vi "odometry_msg.vi"(11 "odometry_msg in":string) -> (2 "Current_Pose":T1, 3 "robot_position_cluster":T2)   [LabVIEW 2014]
uses:
  Robot_Position.ctl
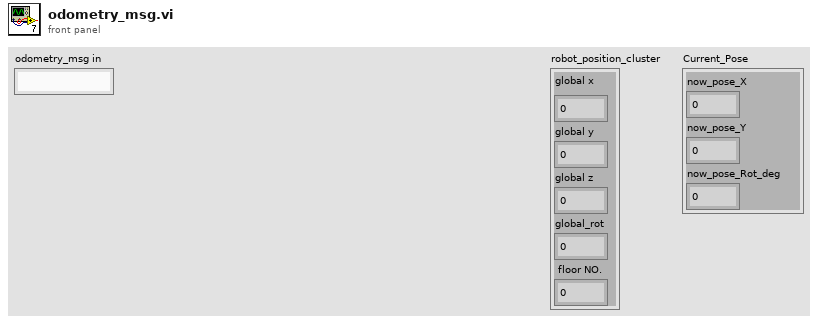
[diagram p1: front panel]
types:
  T1 = cluster{"now_pose_X":dbl, "now_pose_Y":dbl, "now_pose_Rot_deg":dbl}
  T2 = typedef "Robot_Position.ctl" = cluster{"global x":dbl, "global y":dbl, "global z":dbl, "global_rot":dbl, " floor NO.":dbl}
  T3 = cluster{"PoseCovariance":cluster{"Pose":cluster{"Point":cluster{"x":dbl, "y":dbl, "z":dbl}, "Quaternion":cluster{"x":dbl, "y":dbl, "z":dbl, "w":dbl}}, "Covariance":dbl}, "TwistCovariance":cluster{"Twist":cluster{"Linear":cluster{"x":dbl, "y":dbl, "z":dbl}, "Angular":cluster{"x":dbl, "y":dbl, "z":dbl}}, "Covariance":dbl}}
  T4 = cluster{"Roll (y)":dbl, "Pitch(x)":dbl, "Yaw (z)":dbl}
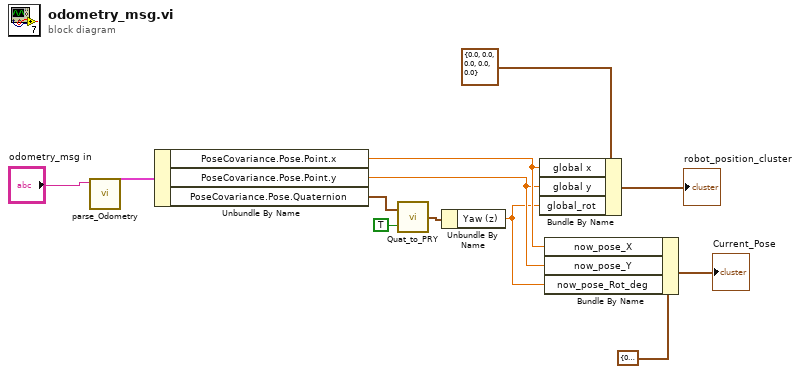
[diagram p0: block diagram]
diagram:
  n1 = call <vilib>:"parse_Odometry.vi"("msg in"="odometry_msg in") -> ("Odometry"=w12:T3)  [unwired: 4 in, 4 out]
  n2 = Unbundle By Name(w12) -> ("PoseCovariance.Pose.Point.x"=w3:dbl, "PoseCovariance.Pose.Point.y"=w2:dbl, "PoseCovariance.Pose.Quaternion"=w11:cluster{"x":dbl, "y":dbl, "z":dbl, "w":dbl})
  n3 = call <vilib>:"Quat_to_PRY.vi"("toDegrees? (T)"=TRUE, "Quaternion"=w11) -> ("Orientation"=w9:T4)
  n4 = Unbundle By Name(w9) -> ("Yaw (z)"=w1:dbl)
  n5 = Bundle By Name(cluster=T2 {"global x"=0.0, "global y"=0.0, "global z"=0.0, "global_rot"=0.0, " floor NO."=0.0} ("robot position"), "global x"=w3, "global y"=w2, "global_rot"=w1) -> (→"robot_position_cluster":T2)
  n6 = Bundle By Name(cluster=T1 {"now_pose_X"=0.0, "now_pose_Y"=0.0, "now_pose_Rot_deg"=0.0} ("Current_Pose"), "now_pose_X"=w3, "now_pose_Y"=w2, "now_pose_Rot_deg"=w1) -> (→"Current_Pose":T1)
